vi "Clear ConvBox.vi"(8 "error in":errorcluster, 10 "address string":string, 11 "VISA resource in":refnum<visa-resource-name>) -> (0 "error out":errorcluster, 1 "ibsta":T1, 3 "VISA resource out":refnum<visa-resource-name>)   [LabVIEW 2018, in "Protocols.lvlib" / "RS-xxx to GPIB ConvBox.lvclass"]
uses:
  RS-xxx to GPIB ConvBox.lvclass
  <vilib>/Instr/_visa.llb/GPIB Status Boolean Array.ctl
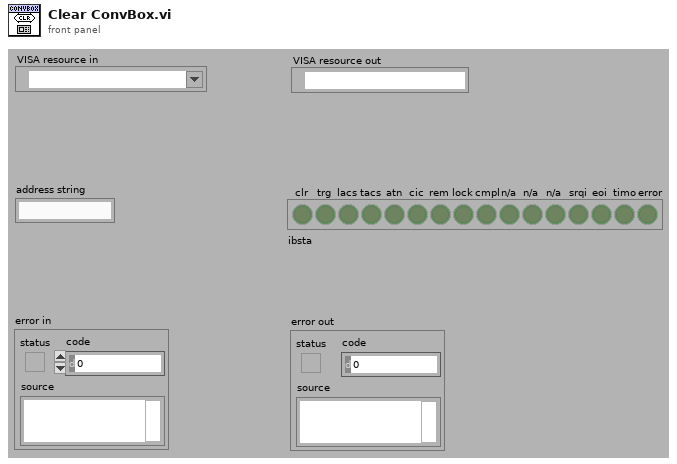
[diagram p1: front panel]
types:
  T1 = typedef "GPIB Status Boolean Array.ctl" = bool[]
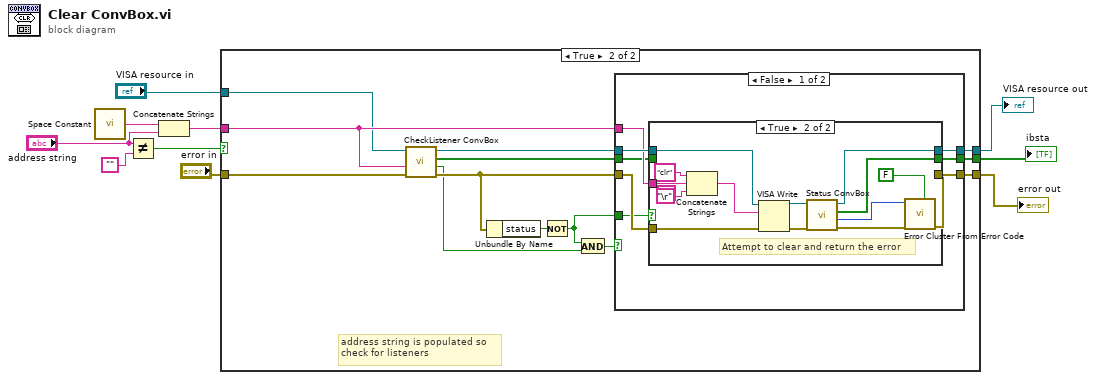
[diagram p0: block diagram]
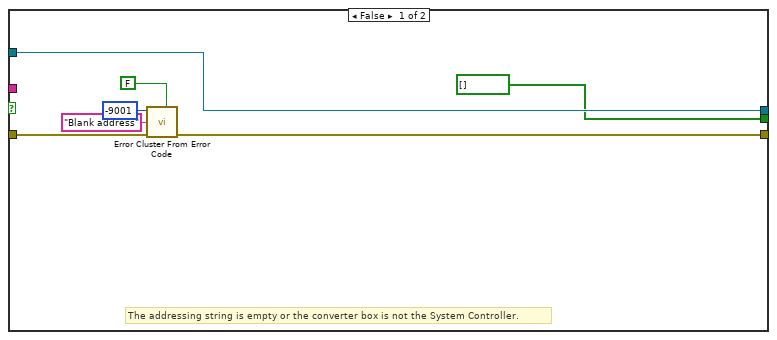
[diagram p2: hidden frame]
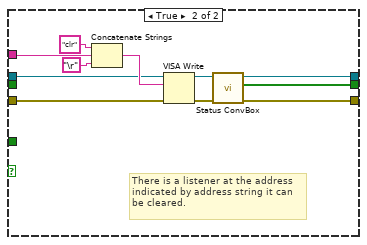
[diagram p4: hidden frame]
diagram:
  n1 = call <vilib>:"Space Constant.vi"() -> ("String"=w10:string)
  n2 = Not Equal?(x="address string", y="") -> (x != y?=w1:bool)
  n3 = Concatenate Strings(w10, "address string") -> (w4:string)
  n4 = case shown="True" w1 {
    tunnel: [w17 w30] -> w7
    tunnel: [T1 [] ("ibsta") w29] -> w6
    tunnel: [w14 w28] -> w5
    tunnel: w4 -> [_ w25]
    tunnel: "error in" -> [w15 w27]
    tunnel: "VISA resource in" -> [w17 w24]
    frame False {
      # "The addressing string is empty or the converter box is not the System Controller."
      n5 = call <vilib>:"Error Cluster From Error Code.vi"("is warning? (False)"=FALSE, "error in (no error)"=w15, "error message (\"\")"="Blank address" ("error message (\"\")"), "error code (0)"=-9001) -> ("error out"=w14:errorcluster)  [unwired: 5 in]
    }
    frame True {
      # "address string is populated so \ncheck for listeners"
      n6 = call "CheckListener ConvBox.vi"("error in"=w27, "address string"=w25, "VISA resource in"=w24) -> ("error out"=w23:errorcluster, "listener found"=w21:bool, "ibsta"=w19:T1, "VISA resource out"=w26:refnum<visa-resource-name>)  [unwired: 5 in]
      n7 = Unbundle By Name(w23) -> ("status"=w20:bool)
      n8 = Not(x=w20) -> (.not. x?=w18:bool)
      n9 = And(x=w18, y=w21) -> (x .and. y?=w22:bool)
      n10 = case shown="False" w22 {
        tunnel: [w35 w66] -> w30
        tunnel: [w34 w65] -> w29
        tunnel: [w38 w64] -> w28
        tunnel: w23 -> [w37 w61]
        tunnel: w26 -> [w36 w57]
        tunnel: w25 -> [w33 w56]
        tunnel: w19 -> [w31 _]
        tunnel: w18 -> [w32 _]
        frame False {
          (unwired) "\r"
          n11 = case shown="True" w32 {
            tunnel: [w39 w54] -> w38
            tunnel: w37 -> [w39 w51]
            tunnel: w36 -> [w40 w47]
            tunnel: [w40 w46] -> w35
            tunnel: [w41 w44] -> w34
            tunnel: w33 -> [_ w43]
            tunnel: w31 -> [w41 _]
            frame False {
              # "Error returned from checklisteners"
            }
            frame True {
              # "Attempt to clear and return the error"
              n12 = Concatenate Strings("clr", w43, "\r") -> (w52:string)
              n13 = VISA Write(VISA resource name=w47, write buffer=w52, error in (no error)=w51) -> (VISA resource name out=w48:refnum<visa-resource-name>, error out=w50:errorcluster)  [unwired: 1 out]
              n14 = call "Status ConvBox.vi"("error in (no error)"=w50, "VISA resource name"=w48) -> ("error out"=w49:errorcluster, "GPIB error"=w45:i16, "ibsta"=w44:T1, "VISA resource out"=w46:refnum<visa-resource-name>)  [unwired: 6 in]
              n15 = call <vilib>:"Error Cluster From Error Code.vi"("is warning? (False)"=FALSE, "error in (no error)"=w49, "error code (0)"=w45) -> ("error out"=w54:errorcluster)  [unwired: 6 in]
            }
          }
        }
        frame True {
          # "There is a listener at the address\nindicated by address string it can\nbe cleared."
          n16 = Concatenate Strings("clr", w56, "\r") -> (w58:string)
          n17 = VISA Write(VISA resource name=w57, write buffer=w58, error in (no error)=w61) -> (VISA resource name out=w63:refnum<visa-resource-name>, error out=w62:errorcluster)  [unwired: 1 out]
          n18 = call "Status ConvBox.vi"("error in (no error)"=w62, "VISA resource name"=w63) -> ("error out"=w64:errorcluster, "ibsta"=w65:T1, "VISA resource out"=w66:refnum<visa-resource-name>)  [unwired: 6 in, 1 out]
        }
      }
    }
  }
  "VISA resource out" <- w7
  "ibsta" <- w6
  "error out" <- w5
